vi "BuildDataSave.vi"(6 "units":string[](array[string]), 7 "varnames":string[](array[string]), 8 "raw data filename string":string, 9 "Steady Indicator":bool=TRUE, 10 "Array":dbl[](array[numeric]), 11 "Saving Cluster":T1) -> ()   [LabVIEW 2017]
doc: "Creates build file of average of raw data file"
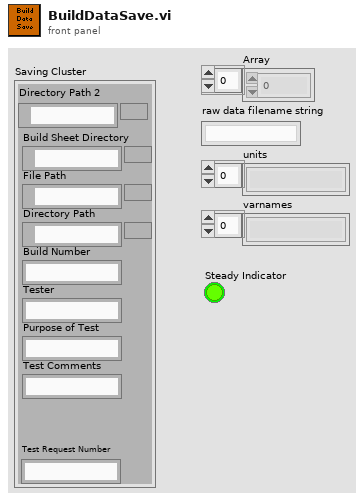
[diagram p1: front panel]
types:
  T1 = cluster{"Build Sheet Directory":path, "File Path":path, "Directory Path":path, "Build Number":string, "Tester":string, "Purpose of Test":string, "Test Comments ":string, "Test Request Number":string, "Directory Path 2":path}
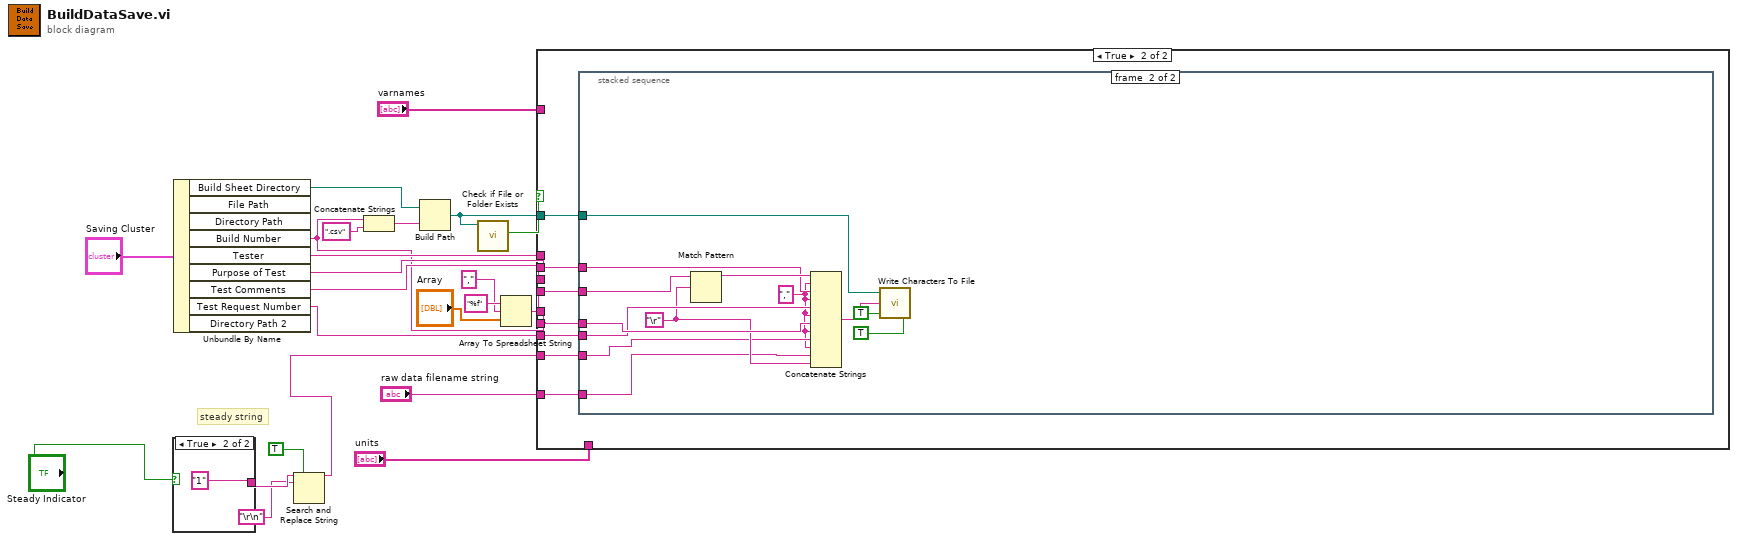
[diagram p0: block diagram]
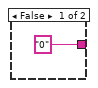
[diagram p2: hidden frame]
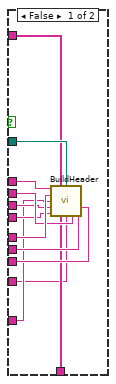
[diagram p3: hidden frame]
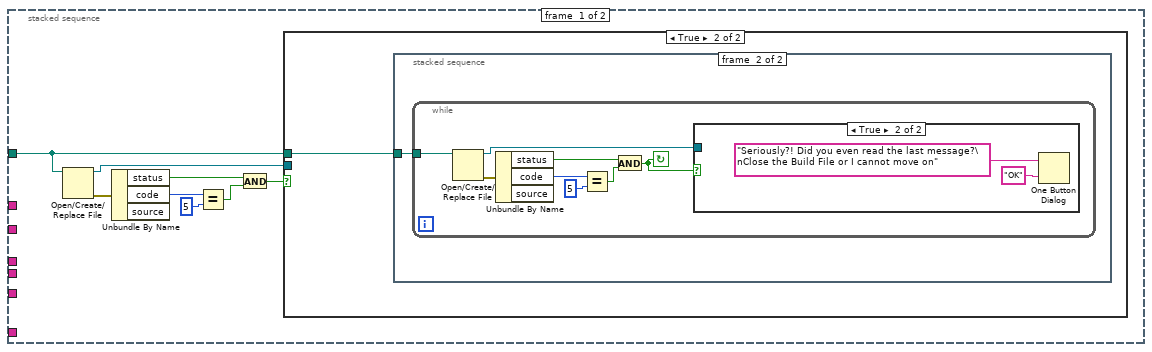
[diagram p4: hidden frame]
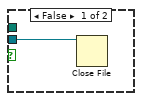
[diagram p5: hidden frame]
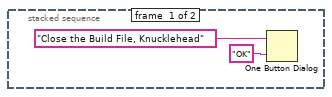
[diagram p6: hidden frame]
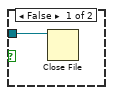
[diagram p7: hidden frame]
diagram:
  # "steady string"
  n1 = case shown="True" "Steady Indicator" {
    tunnel: ["0" "1"] -> w4
    frame False {
    }
    frame True {
    }
  }
  n2 = Unbundle By Name("Saving Cluster") -> ("Build Sheet Directory"=w20:path, "Build Number"=w9:string, "Tester"=w18:string, "Purpose of Test"=w17:string, "Test Comments"=w16:string, "Test Request Number"=w10:string)  [unwired: 3 out]
  n3 = Search and Replace String(replace all?=TRUE ("replace all? (F)"), input string=w4, search string="\r\n") -> (result string=w1:string)  [unwired: 5 in, 3 out]
  n4 = Concatenate Strings(w9, ".csv" ("string")) -> (w21:string)
  n5 = Build Path(base path=w20, name or relative path=w21) -> (appended path=w19:path)
  n6 = call <vilib>:"Check if File or Folder Exists.vi"("path"=w19) -> ("file or folder exists?"=w11:bool)  [unwired: 8 in, 2 out]
  n7 = Array To Spreadsheet String(delimiter (Tab)=",", array="Array", 3:"%f" ("format string")) -> (spreadsheet string=w12:string)
  n8 = case shown="True" w11 {
    tunnel: w19 -> [w32 w44]
    tunnel: w9 -> [w37 _]
    tunnel: w18 -> [w36 _]
    tunnel: w17 -> [w35 w42]
    tunnel: w16 -> [w34 _]
    tunnel: w12 -> [w33 w43]
    tunnel: w10 -> [w31 w41]
    tunnel: w9 -> [w30 w40]
    tunnel: "raw data filename string" -> [w27 w39]
    tunnel: "units" -> [w29 _]
    tunnel: "varnames" -> [w28 _]
    tunnel: w1 -> [w26 w38]
    frame False {
      n9 = call "BuildHeader.vi"("Tester"=w36, "varnames"=w28, "Build Sheet File Path"=w32, "Build Name"=w37, "raw data filename"=w27, "Comments on Test"=w34, "Build Number"=w31, "Spreadsheet Data"=w33, "units"=w29, "steady string"=w26, "Purpose of Test"=w35, "Test Request Number"=w30) -> ()  [unwired: 3 in, 1 out]
    }
    frame True {
      n10 = stacked-sequence {
        tunnel: w44 -> [w52 w75]
        tunnel: w43 -> [_ w81]
        tunnel: w42 -> [_ w79]
        tunnel: w41 -> [_ w73]
        tunnel: w40 -> [_ w74]
        tunnel: w39 -> [_ w71]
        tunnel: w38 -> [_ w70]
        frame #0 {
          n11 = Open/Create/Replace File(file path (use dialog)=w52) -> (refnum out=w51:refnum<file>, error out=w50:errorcluster)  [unwired: 5 in, 1 out]
          n12 = Unbundle By Name(w50) -> ("status"=w46:bool, "code"=w49:i32)  [unwired: 1 out]
          n13 = Equal?(x=w49, y=5) -> (x = y?=w47:bool)
          n14 = And(x=w46, y=w47) -> (x .and. y?=w45:bool)
          n15 = case shown="True" w45 {
            tunnel: w52 -> [_ w54]
            tunnel: w51 -> [w53 _]
            frame False {
              n16 = Close File(refnum=w53) -> ()  [unwired: 1 in, 2 out]
            }
            frame True {
              n17 = stacked-sequence {
                tunnel: w54 -> [_ w57]
                frame #0 {
                  n18 = One Button Dialog(message="Close the Build File, Knucklehead", button name ("OK")="OK") -> ()  [unwired: 1 out]
                }
                frame #1 {
                  n19 = while {
                    tunnel: w57 -> [w61]
                    stop <- w58 continue-if-true
                    n20 = Open/Create/Replace File(file path (use dialog)=w61) -> (refnum out=w60:refnum<file>, error out=w65:errorcluster)  [unwired: 5 in, 1 out]
                    n21 = Unbundle By Name(w65) -> ("status"=w63:bool, "code"=w59:i32)  [unwired: 1 out]
                    n22 = Equal?(x=w59, y=5) -> (x = y?=w62:bool)
                    n23 = And(x=w63, y=w62) -> (x .and. y?=w58:bool)
                    n24 = case shown="True" w58 {
                      tunnel: w60 -> [w66 _]
                      frame False {
                        n25 = Close File(refnum=w66) -> ()  [unwired: 1 in, 2 out]
                      }
                      frame True {
                        n26 = One Button Dialog(message="Seriously?! Did you even read the last message?\nClose the Build File or I cannot move on", button name ("OK")="OK") -> ()  [unwired: 1 out]
                      }
                    }
                  }
                }
              }
            }
          }
        }
        frame #1 {
          w69 = "," ("string")
          w72 = "\r"
          n27 = Match Pattern(string=w81, regular expression=w72) -> (before substring=w80:string)  [unwired: 1 in, 3 out]
          n28 = Concatenate Strings(w80, w69, w79, w69, w73, w69, w74, w69, w70, w69, w71, w72) -> (w78:string)
          n29 = call <vilib>:"Write Characters To File.vi"("convert eol? (no:F)"=TRUE, "append to file? (new file:F)"=TRUE, "character string"=w78, "file path (dialog if empty)"=w75) -> ()  [unwired: 1 in, 1 out]
        }
      }
    }
  }
